vi "FTW-Producer-Construct.vi"(5 "Server Address":string, 7 "Identity":string, 9 "Buffer Depth (1)":i32=1, 11 "error in":errorcluster) -> (4 "FTW-Producer Out":refnum<class "FTW-Producer.lvclass">, 15 "error out":errorcluster)   [LabVIEW 2015, in "FTW-Producer.lvclass"]
uses:
  FTW-Producer.lvclass
  Ether/FTW-Ether-EndpointType.ctl
  FTW-Producer.lvclass/FTW-Producer.ctl
  Endpoint/FTW-Endpoint.lvclass
  Ether/FTW-Ether.lvclass
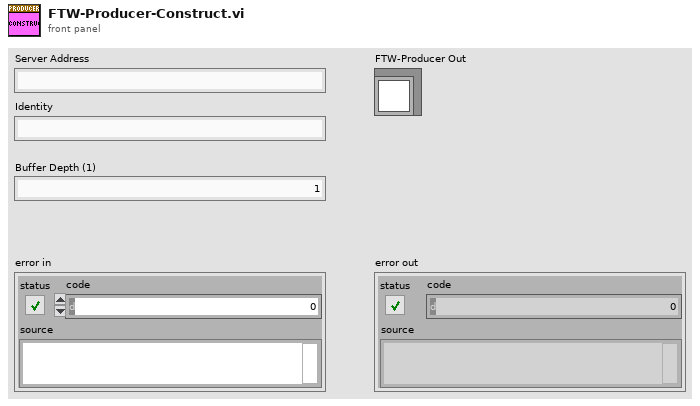
[diagram p1: front panel]
types:
  T1 = typedef "FTW-Ether.lvclass/FTW-Ether-EndpointType.ctl" = enum16{"Server", "Client", "Publisher", "Subscriber"}
  T2 = typedef "FTW-Ether.lvclass/FTW-Ether-MessageTransportScheme.ctl" = enum16{"In process (inproc://)", "TCP (tcp://)"}
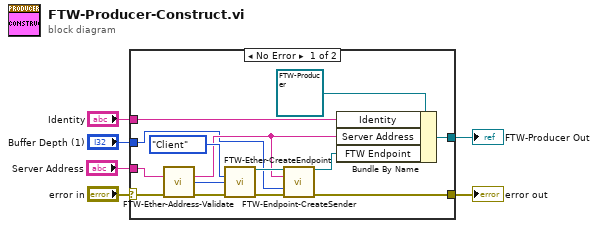
[diagram p0: block diagram]
diagram:
  n1 = case shown="No Error" "error in" {
    selector: "error in" -> [w18 w21]
    tunnel: [w11 w21] -> w4
    tunnel: [w19 _] -> w6
    tunnel: "Server Address" -> [w14 _]
    tunnel: "Identity" -> [w12 _]
    tunnel: "Buffer Depth (1)" -> [w7 _]
    frame No Error {
      n2 = call "FTW-Ether-Address-Validate.vi"("Address"=w14, "error in"=w18) -> ("Sanitized Address"=w8:string, "Message Transport Scheme"=w15:T2, "error out"=w17:errorcluster)  [unwired: 11 in]
      n3 = call "FTW-Ether-CreateEndpoint.vi"("Endpoint Type"=FTW-Ether-EndpointType."Client", "Message Transport Scheme"=w15, "error in"=w17) -> ("FTW Endpoint"=w10:refnum<class "FTW-Endpoint.lvclass">, "error out"=w13:errorcluster)  [unwired: 11 in]
      n4 = call-dynamic "FTW-Endpoint-CreateSender.vi"("FTW Endpoint"=w10, "Endpoint Address"=w8, "Buffer Depth (1)"=w7, "error in"=w13) -> ("FTW Endpoint out"=w9:refnum<class "FTW-Endpoint.lvclass">, "error out"=w11:errorcluster)  [unwired: 10 in]
      n5 = Bundle By Name(cluster=refnum<class "FTW-Producer.lvclass"> refnum ("LVmsg_Client in"), "Identity"=w12, "Server Address"=w8, "FTW Endpoint"=w9) -> (w19:refnum<class "FTW-Producer.lvclass">)
    }
    frame Error {
    }
  }
  "FTW-Producer Out" <- w6
  "error out" <- w4
